vi "Get Keyboard Locking Status.vi"(4 "error in (no error)":errorcluster, 7 "VISA resource name":refnum<visa-resource-name>) -> (0 "error out":errorcluster, 2 "Lock Option":T1(ring), 3 "VISA resource name out":refnum<visa-resource-name>)   [LabVIEW 2018, in "Newport ESP301.lvlib"]
doc: "Get lock / unlock status of the keyboard of ESP301."
uses:
  Newport ESP301.lvlib
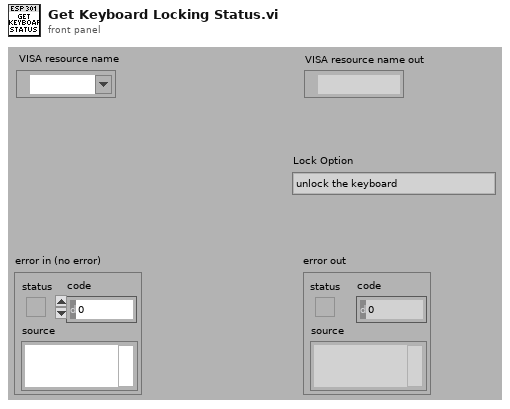
[diagram p1: front panel]
types:
  T1 = enum16{"unlock the keyboard", "lock all buttons but the “Motor ON/OFF”", "lock all buttons"}
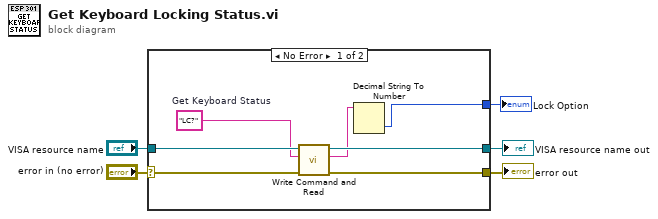
[diagram p0: block diagram]
diagram:
  n1 = case shown="No Error" "error in (no error)" {
    selector: "error in (no error)" -> [w11 w14]
    tunnel: [w9 w14] -> w4
    tunnel: "VISA resource name" -> [w12 w13]
    tunnel: [w10 w13] -> w2
    tunnel: [w6 _] -> w1
    frame No Error {
      w7 = "LC?"  # Get Keyboard Status
      n2 = call "Write Command and Read.vi"("error in (no error)"=w11, "Command"=w7, "VISA resource name"=w12) -> ("error out"=w9:errorcluster, "Returned string"=w8:string, "VISA resource name out"=w10:refnum<visa-resource-name>)  [unwired: 4 in]
      n3 = Decimal String To Number(string=w8) -> (number=w6:i32)  [unwired: 2 in, 1 out]
    }
    frame Error {
    }
  }
  "error out" <- w4
  "VISA resource name out" <- w2
  "Lock Option" <- w1
